vi "Get SMO Serial Number.vi"(8 "error in (no error)":errorcluster, 11 "instrument.PPMS in":refnum<class "instrument.PPMS.lvclass">) -> (0 "error out":errorcluster, 2 "Serial Number":string, 3 "instrument.PPMS out":refnum<class "instrument.PPMS.lvclass">)   [LabVIEW 2019, in "instrument.PPMS.lvclass"]
doc: "Override this VI to return the serial number of your Instrument"
uses:
  instrument.PPMS.lvclass
  <userlib>/LevyLab/Instrument Framework/Instrument Types/Cryostat/Instrument.Cryostat.lvclass
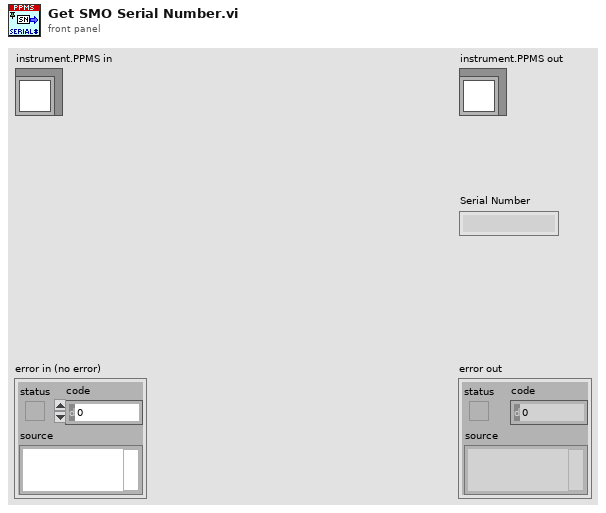
[diagram p1: front panel]
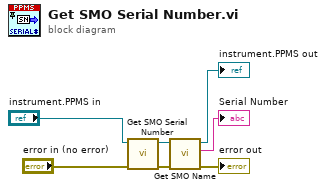
[diagram p0: block diagram]
diagram:
  n1 = call-parent "Get SMO Serial Number.vi"("error in (no error)"="error in (no error)", "Instrument in"="instrument.PPMS in") -> ("error out"=w5:errorcluster, "Instrument out"=w2:refnum<class "instrument.PPMS.lvclass">)  [unwired: 7 in, 1 out]
  n2 = call-dynamic "Get SMO Name.vi"("error in (no error)"=w5, "instrument.PPMS in"=w2) -> ("error out"=→"error out":errorcluster, "SMO Name"=→"Serial Number":string, "instrument.PPMS out"=→"instrument.PPMS out":refnum<class "instrument.PPMS.lvclass">)  [unwired: 7 in]
